vi "Read Attribute Notes.vi"(11 "Sequence Dialog in":refnum<class "TestStep Edit Dialog.lvclass">) -> (2 "Attribute Notes":string[](array[string]), 3 "Sequence Dialog out":refnum<class "TestStep Edit Dialog.lvclass">)   [LabVIEW 2017, in "TestStep Edit Dialog.lvclass"]
uses:
  TestStep Edit Dialog.lvclass
  TestStep Edit Dialog.lvclass/TestStep Edit Dialog.ctl
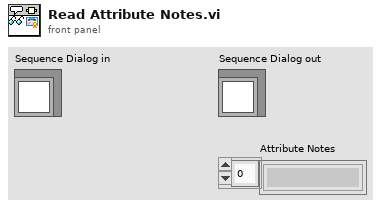
[diagram p1: front panel]
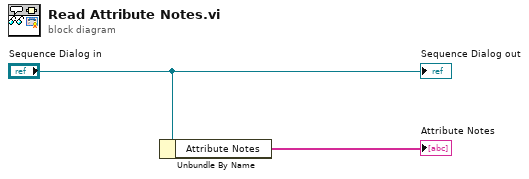
[diagram p0: block diagram]
diagram:
  n1 = Unbundle By Name("Sequence Dialog in") -> ("Attribute Notes"=→"Attribute Notes":string[])
  "Sequence Dialog out" <- "Sequence Dialog in"
